vi "FT_Purge.vi"(1 "Purge Flags":u32(ring)=3 items=["FT_PURGE_RX"=1, "FT_PURGE_TX"=2, "FT_PURGE_RX | FT_PURGE_TX"=3], 2 "Handle":u32) -> (0 "FT_Status":u32)   [LabVIEW 2017]
uses:
  FTD2XX.dll
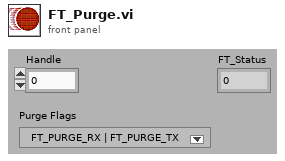
[diagram p1: front panel]
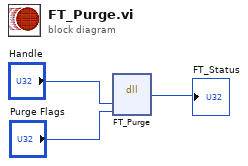
[diagram p0: block diagram]
diagram:
  n1 = dll-call lib="FTD2XX.dll" fn="FT_Purge"("Handle"="Handle", "Flags"="Purge Flags") -> ("FT_Status"=→"FT_Status":u32)  [unwired: 5 in, 2 out]
